vi "Flatten Value.vi"(8 "error in (no error)":errorcluster, 11 "Boolean in":refnum<class "Persistence.lvclass">) -> (0 "error out":errorcluster, 2 "Value":string, 3 "Boolean out":refnum<class "Persistence.lvclass">)   [LabVIEW 2017, in "Custom Type Test Executive.lvlib" / "Persistence.lvclass"]
uses:
  <vilib>/gpm_packages/@cs/test-executive/Source/Custom Type Test Executive/Persistence Data Type/Persistence.lvclass
  <vilib>/gpm_packages/@cs/test-executive/Source/Custom Type Test Executive/Persistence Data Type/Persistence.lvclass/Persistence.ctl
  <vilib>/gpm_packages/@cs/persistence/source/IPersist/IPersist.lvclass
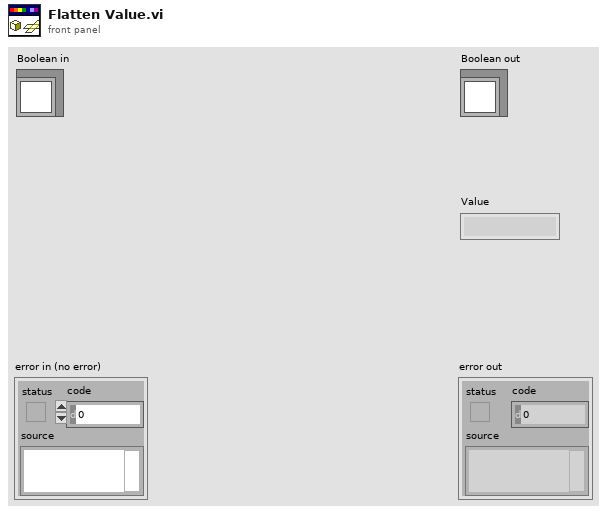
[diagram p1: front panel]
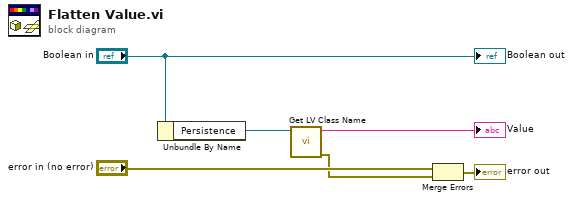
[diagram p0: block diagram]
diagram:
  n1 = Unbundle By Name("Boolean in") -> ("Persistence"=w3:refnum<class "IPersist.lvclass">)
  n2 = call <vilib>:"Get LV Class Name.vi"("object"=w3) -> ("error out"=w1:errorcluster, "class name"=→"Value":string)  [unwired: 9 in]
  n3 = Merge Errors("error in (no error)", w1) -> (→"error out":errorcluster)
  "Boolean out" <- "Boolean in"
